vi "GEA2_Read_ERD.vi"(0 "session in":refnum<k35>, 7 "dst":i64 format="%x", 9 "ERD":i64 format="%x", 11 "error in (no error)":errorcluster) -> (4 "session out":refnum<k35>, 6 "Raw Data":string, 8 "Read ERD":T1 {"ERD Number" format="%x"}, 15 "error out":errorcluster)   [LabVIEW 2021]
uses:
  Controles/Read_ERD.ctl
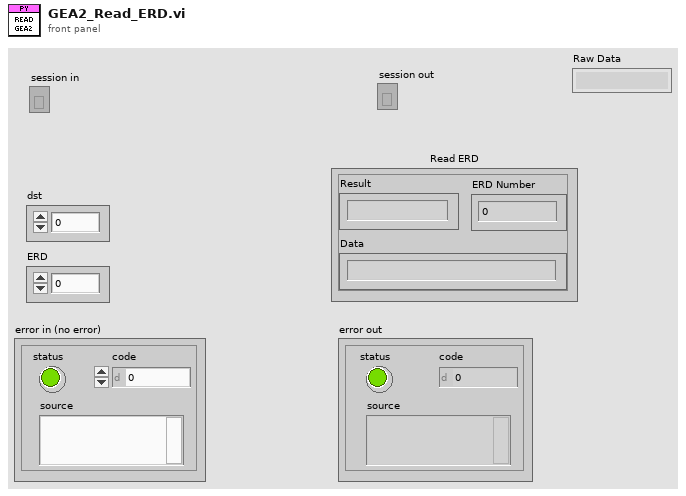
[diagram p1: front panel]
types:
  T1 = typedef "Read_ERD.ctl" = cluster{"Result":string, "ERD Number":i64, "Data":string}
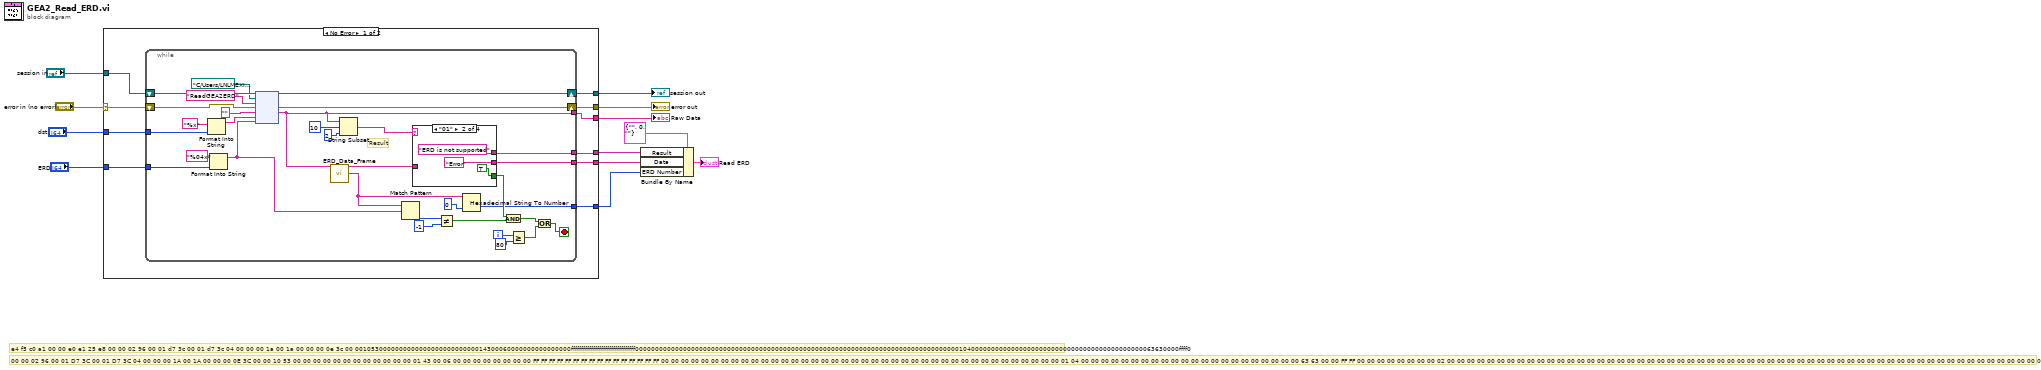
[diagram p0: block diagram]
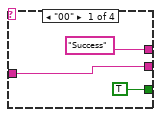
[diagram p2: hidden frame]
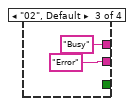
[diagram p3: hidden frame]
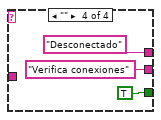
[diagram p4: hidden frame]
diagram:
  # "00 00 02 96 00 01 D7 3C 00 01 D7 3C 04 00 00 00 1A 00 1A 00 00 00 0E 3C 00 00 10 53 00 00 00 00 00 00 00 00 00 00 00 00 01 43 00 06 00 00 00 00 00 00 00 00 FF FF FF FF FF FF FF FF FF FF FF FF FF FF FF FF 00 00 00 00 00 00 00 00 00 00 00 00 00 00 00 00 00 00 00 00 00 00 00 00 00 00 00 00 00 00 00 00 00 00 00 00 00 00 00 00 01 04 00 00 00 00 00 00 00 00 00 00 00 00 00 00 00 00 00 00 00 00 00 00 63 63 00 00 FF FF 00 00 00 00 00 00 00 00 02 00 00 00 00 00 00 00 00 00 00 00 00 00 00 00 00 00 00 00 00 00 00 00 00 00 00 00 00 00 00 00 00 00 00 00 00 00 00 00 00 00 00 00 00 00 00 00 00 00 00 00 00 00 00 00 00 00 00 00 00 00 00 00 00 00 00 00 00 00 00 00 00 00 00 00 00 00 00 00 00 00 00 00 00 00"
  # "e4 f5 c0 a1 00 00 e0 e1 25 e8 00 00 02 96 00 01 d7 3c 00 01 d7 3c 04 00 00 00 1a 00 1a 00 00 00 0e 3c 00 001053000000000000000000000000014300060000000000000000ffffffffffffffffffffffffffffffff0000000000000000000000000000000000000000000000000000000000000000000000000000000001040000000000000000000000000000000000000000000063630000ffff0"
  n1 = case shown="No Error" "error in (no error)" {
    selector: "error in (no error)" -> [w17 w67]
    tunnel: "dst" -> [w22 _]
    tunnel: "ERD" -> [w15 _]
    tunnel: "session in" -> [w21 w66]
    tunnel: [w20 w66] -> w9
    tunnel: [w19 w67] -> w8
    tunnel: [w18 _] -> w7
    tunnel: [w16 _] -> w3
    tunnel: [w14 _] -> w2
    tunnel: [w13 _] -> w1
    frame No Error {
      n2 = while {
        tunnel: w22 -> [w54]
        tunnel: [w50] -> w18
        tunnel: [w39] -> w16
        tunnel: w15 -> [w38]
        shift-right: [w52] -> w20
        shift-left: w21 -> [w53]
        shift-right: [w51] -> w19
        shift-left: w17 -> [w40]
        tunnel: [w31] -> w14
        tunnel: [w23] -> w13
        i -> [w26]
        stop <- w28 stop-if-true
        # "Result"
        n3 = Format Into String(format string="%x", w54) -> (resulting string=w46:string)  [unwired: 2 in, 1 out]
        n4 = Format Into String(format string="%04x", w38) -> (resulting string=w35:string)  [unwired: 2 in, 1 out]
        n5 = node(w53, path "C:/Users/LNLMEXID/Desktop/GEA3 Python/Main.py" ("module path"), "ReadGEA2ERD" ("function name"), w40, "" ("data_hex"), w46, w35) -> (w52:refnum<k35>, w51:errorcluster, w23:string)  [unwired: 2 in, 2 out]
        n6 = call "ERD_Data_Frame.vi"("Frame"=w23) -> ("Data"=w32:string, "ERD"=w30:string)  [unwired: 13 in]
        n7 = String Subset(string=w23, offset (0)=10, length (rest)=2 ("length (rest)")) -> (substring=w42:string)
        n8 = Match Pattern(string=w30, regular expression=w35) -> (offset past match=w37:i32)  [unwired: 1 in, 3 out]
        n9 = case shown="\"01\"" w42 {
          tunnel: ["Success" "ERD is not supported" "Busy" "Desconectado"] -> w50
          tunnel: w32 -> [w56 _ _ _]
          tunnel: [w56 "Error" "Error" "Verifica conexiones"] -> w39
          tunnel: [TRUE TRUE _ TRUE] -> w33
          frame "00" {
          }
          frame "01" {
          }
          frame "02", Default {
          }
          frame "" {
          }
        }
        n10 = Not Equal?(x=w37, y=-1) -> (x != y?=w34:bool)
        n11 = Hexadecimal String To Number(string=w30, default (0uL)=i64 0 ("ERD Number")) -> (number=w31:i64)  [unwired: 1 in, 1 out]
        n12 = And(x=w33, y=w34) -> (x .and. y?=w27:bool)
        n13 = Greater Or Equal?(x=w26, y=80) -> (x >= y?=w24:bool)
        n14 = Or(x=w27, y=w24) -> (x .or. y?=w28:bool)
      }
    }
    frame Error {
    }
  }
  "session out" <- w9
  "error out" <- w8
  "Raw Data" <- w1
  n15 = Bundle By Name(cluster=T1 {"Result"="", "ERD Number"=0, "Data"=""} ("Read ERD"), "Result"=w7, "Data"=w3, "ERD Number"=w2) -> (→"Read ERD":T1)
